vi "GlobalWriteFile.vi"() -> ()   [LabVIEW 2022 SP3]
panel:
  out "Path":path
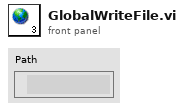
[diagram p1: front panel]
diagram:
